vi "Remove Package from Feed.vi"(8 "error in":errorcluster, 9 "delete package file? (F)":bool, 10 "package filename":string, 11 "feed folderpath in":path) -> (0 "error out":errorcluster, 1 "package file deleted":bool, 2 "removed package filepath":path, 3 "feed folderpath out":path)   [LabVIEW 2014, in "NIPM_API.lvlib"]
doc: "Removes a package from a feed\n\nINPUT(s)\n<B>Feed folderpath</B>: Specifies the folder containing the feed\n\n<B>Package filename</B>: Specifies the filename of the package to be removed from the feed\n\n<B>Delete package file?</B>: If this input is set to TRUE, this VI will delete the package file (.nipkg) in the feed folderpath after removing the package from the feed. If this input is set to FALSE, the package file (.nipkg) will remain in the feed folderpath after removing the package from the feed.\n\nOUTPUT(s)\n<B>Feed folderpath out</B>: Outputs the specified feed folderpath\n\n<B>Removed package filepath</B>: Outputs the filepath of the package that was removed from the feed\n\n<B>Package file deleted</B>: Outputs whether this VI successfully deleted the package file (.nipkg) in the feed folderpath"
uses:
  NIPM_API.lvlib
  _support/Version Comparison Operator.ctl
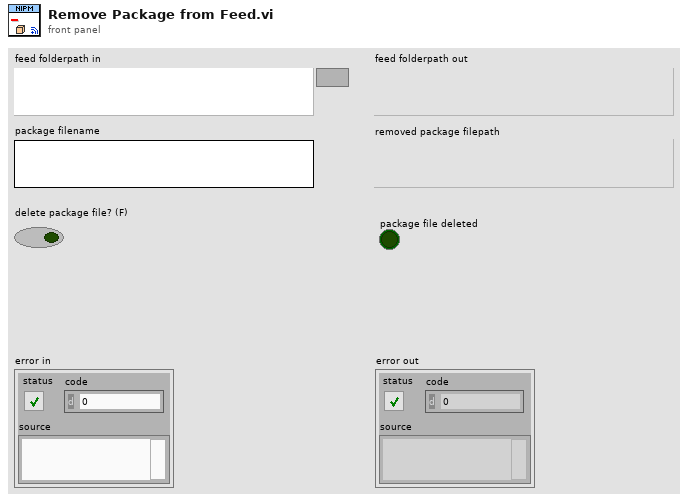
[diagram p1: front panel]
types:
  T1 = typedef "NIPM_API.lvlib/Version Comparison Operator.ctl" = enum16{">", ">=", "=", "!=", "<=", "<"}
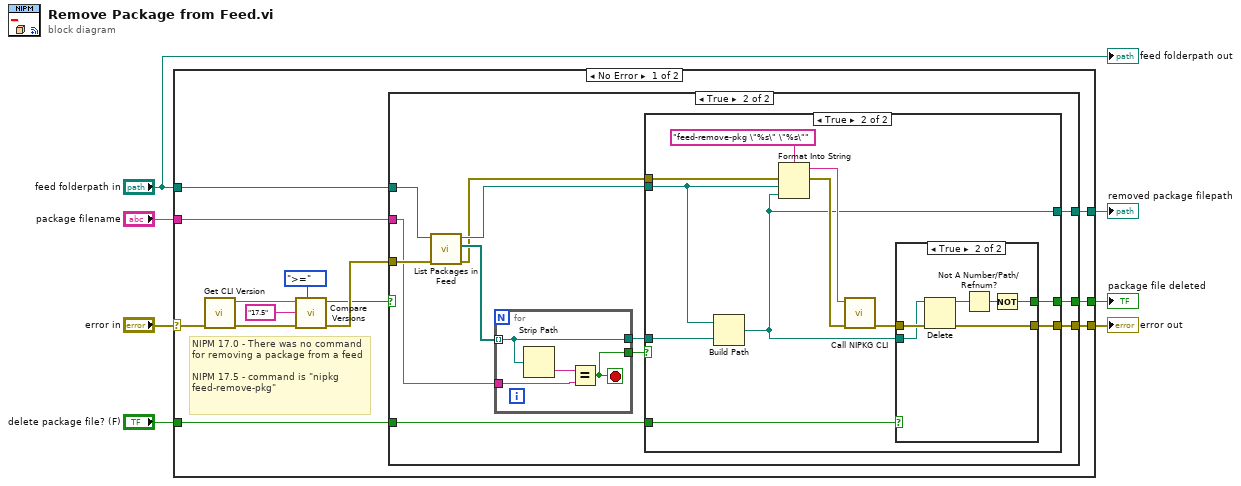
[diagram p0: block diagram]
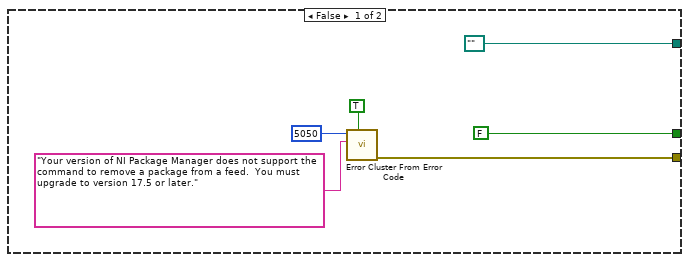
[diagram p2: hidden frame]
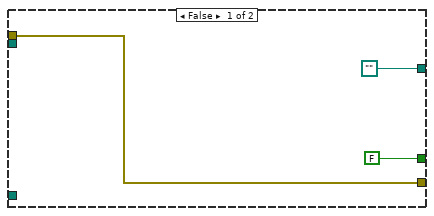
[diagram p3: hidden frame]
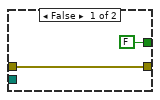
[diagram p4: hidden frame]
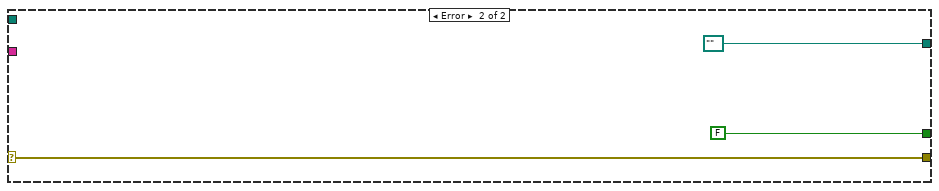
[diagram p5: hidden frame]
diagram:
  n1 = case shown="No Error" "error in" {
    selector: "error in" -> [w17 w67]
    tunnel: [w20 w67] -> w7
    tunnel: "feed folderpath in" -> [w19 _]
    tunnel: "package filename" -> [w18 _]
    tunnel: [w10 path "" ("appended path")] -> w3
    tunnel: "delete package file? (F)" -> [w9 _]
    tunnel: [w8 FALSE] -> w1
    frame No Error {
      # "NIPM 17.0 - There was no command for removing a package from a feed\n\nNIPM 17.5 - command is \"nipkg feed-remove-pkg\""
      n2 = call "Get CLI Version.vi"("error in"=w17) -> ("error out"=w13:errorcluster, "full version string"=w14:string)  [unwired: 9 in]
      n3 = call "Compare Versions.vi"("operator"=Version_Comparison_Operator.">=", "error in"=w13, "version y"="17.5", "version x"=w14) -> ("error out"=w12:errorcluster, "Satisfied?"=w11:bool)  [unwired: 6 in]
      n4 = case shown="True" w11 {
        tunnel: [w21 w37] -> w20
        tunnel: w19 -> [_ w33]
        tunnel: w18 -> [_ w30]
        tunnel: w12 -> [_ w34]
        tunnel: [path "" ("appended path") w36] -> w10
        tunnel: w9 -> [_ w38]
        tunnel: [FALSE w35] -> w8
        frame False {
          n5 = call <vilib>:"Error Cluster From Error Code.vi"("show call chain? (False)"=TRUE, "error message (\"\")"="Your version of NI Package Manager does not support the command to remove a package from a feed.  You must upgrade to version 17.5 or later.", "error code (0)"=5050) -> ("error out"=w21:errorcluster)  [unwired: 6 in]
        }
        frame True {
          n6 = call "List Packages in Feed.vi"("error in"=w34, "feed folderpath in"=w33) -> ("error out"=w28:errorcluster, "package relative filepaths"=w31:path[], "feed folderpath out"=w32:path)  [unwired: 6 in, 1 out]
          n7 = for {
            tunnel: w31 -> [w64] mode=indexing
            tunnel: w30 -> [w62]
            tunnel: [w64] -> w29
            tunnel: [w61] -> w27
            stop <- w61 stop-if-true
            n8 = Strip Path(path=w64) -> (name=w63:string)  [unwired: 1 out]
            n9 = Equal?(x=w63, y=w62) -> (x = y?=w61:bool)
          }
          n10 = case shown="True" w27 {
            tunnel: w38 -> [_ w49]
            tunnel: [w39 w47] -> w37
            tunnel: [path "" w42] -> w36
            tunnel: [FALSE w46] -> w35
            tunnel: w32 -> [_ w44]
            tunnel: w29 -> [_ w43]
            tunnel: w28 -> [w39 w45]
            frame False {
            }
            frame True {
              n11 = Build Path(base path=w44, name or relative path=w43) -> (appended path=w42:path)
              n12 = Format Into String(format string="feed-remove-pkg \"%s\" \"%s\"", error in=w45, w44, w42) -> (resulting string=w51:string, error out=w50:errorcluster)  [unwired: 1 in]
              n13 = call "Call NIPKG CLI.vi"("error in (no error)"=w50, "command"=w51) -> ("error out"=w48:errorcluster)  [unwired: 8 in, 1 out]
              n14 = case shown="True" w49 {
                tunnel: w48 -> [w53 w60]
                tunnel: [w53 w59] -> w47
                tunnel: w42 -> [_ w56]
                tunnel: [FALSE w57] -> w46
                frame False {
                }
                frame True {
                  n15 = Delete(path (use dialog)=w56, error in=w60) -> (deleted path=w55:path, error out=w59:errorcluster)  [unwired: 3 in, 1 out]
                  n16 = Not A Number/Path/Refnum?(number/path/refnum=w55) -> (NaN/Path/Refnum?=w58:bool)
                  n17 = Not(x=w58) -> (.not. x?=w57:bool)
                }
              }
            }
          }
        }
      }
    }
    frame Error {
    }
  }
  "error out" <- w7
  "removed package filepath" <- w3
  "package file deleted" <- w1
  "feed folderpath out" <- "feed folderpath in"
